vi "AT Is Read Only A.vi"(8 "error in (no error)":errorcluster, 10 "Feature":string, 11 "handle":i32) -> (0 "error out":errorcluster, 2 "ReadOnly":bool, 3 "Status":i32)   [LabVIEW 2009]
doc: "Is Read Only\n\nOutput:\n I32 Status\n Bool ReadOnly\n\nInput:\n I32 Handle\n String Feature\n\nThis function can be used to determine whether the feature specified by the Feature parameter can be\nmodified. On return the ReadOnly parameter will contain the value FALSE or TRUE. In the case that\nthe feature can be modified the value of ReadOnly will be TRUE, otherwise it will be FALSE."
uses:
  atcoreA.dll
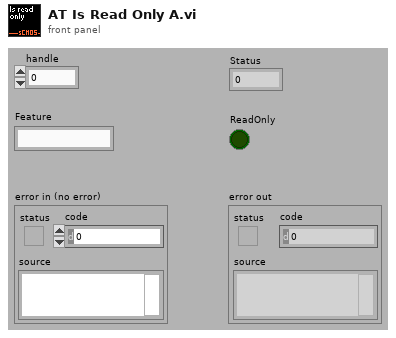
[diagram p1: front panel]
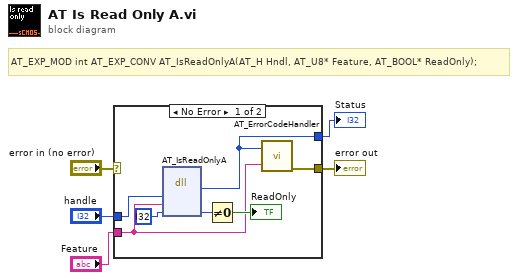
[diagram p0: block diagram]
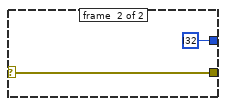
[diagram p2: hidden frame]
diagram:
  # "AT_EXP_MOD int AT_EXP_CONV AT_IsReadOnlyA(AT_H Hndl, AT_U8* Feature, AT_BOOL* ReadOnly);"
  n1 = case shown="No Error" "error in (no error)" {
    selector: "error in (no error)" -> [_ w14]
    tunnel: [w7 i32 ?] -> w5
    tunnel: "handle" -> [w12 _]
    tunnel: "Feature" -> [w6 _]
    tunnel: [w8 w14] -> w1
    frame #0 {
      n2 = dll-call lib="atcoreA.dll" fn="AT_IsReadOnlyA"("Handle"=w12, "Feature"=w6, "ReadOnly"=i32 ?) -> ("Status"=w7:i32, "ReadOnly"=w9:i32)  [unwired: 5 in, 2 out]
      n3 = Not Equal To 0?(x=w9) -> (x != 0?=→"ReadOnly":bool)
      n4 = call "AT_ErrorCodeHandler.vi"("Error"=w7, "Feature Name"=w6) -> ("error out"=w8:errorcluster)  [unwired: 5 in]
    }
    frame #1 {
    }
  }
  "Status" <- w5
  "error out" <- w1
